vi "Vista superior.vi"() -> ()   [LabVIEW 2024]
uses:
  Lamborghini.v2.ctl
  Tsuru.ctl
  Enum. Estarcionar.ctl
  <vilib>/Utility/miscctls.llb/LVPositionTypeDef.ctl
panel:
  out "Retroceder 2":bool
  out "Estacionarse 2":bool
  out "Estacionarse":bool
  out "Retroceder":bool
  in  "Aparecer carro":bool
  in  "Carro":i32
  in  "F1 Auto":T1
  out "Pluma 3":u8(slide)
  out "Led 2":bool
  in  "Stop Button 3":bool
  in  "Tsuru":T2
  out "Pluma 2":u8(slide)
  out "Led 0":bool
  in  "Stop Button 2":bool
  in  "Lamborghini":T3
  out "Led 1":bool
  in  "Stop Button":bool
  out "Pluma":u8(slide)
  # "En el punto de la pluma se debe ver la\nanimación de la pluma levantándose."
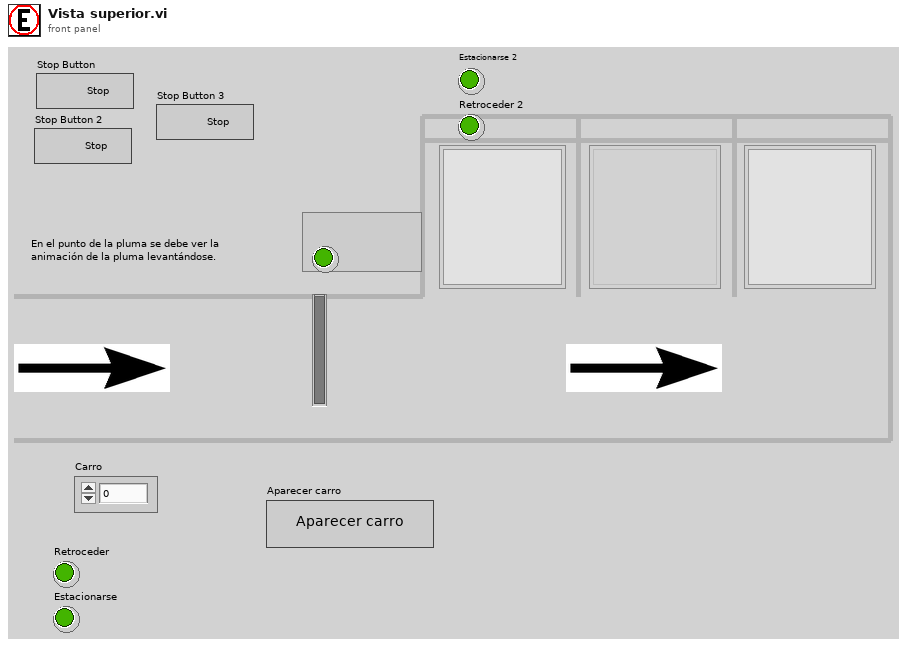
[diagram p1: front panel]
types:
  T1 = typedef "Fórmula 1.ctl" = u16
  T2 = typedef "Tsuru.ctl" = u16
  T3 = typedef "Lamborghini.v2.ctl" = u16
  T4 = typedef "Enum. Estarcionar.ctl" = enum16{"Llegar", "Acceso", "Retroceder", "Animación", "Pluma", "Avanzar", "Girar", "Estacionar", "No hacer nada"}
  T5 = typedef "LVPositionTypeDef.ctl" = cluster{"Left":i32, "Top":i32}
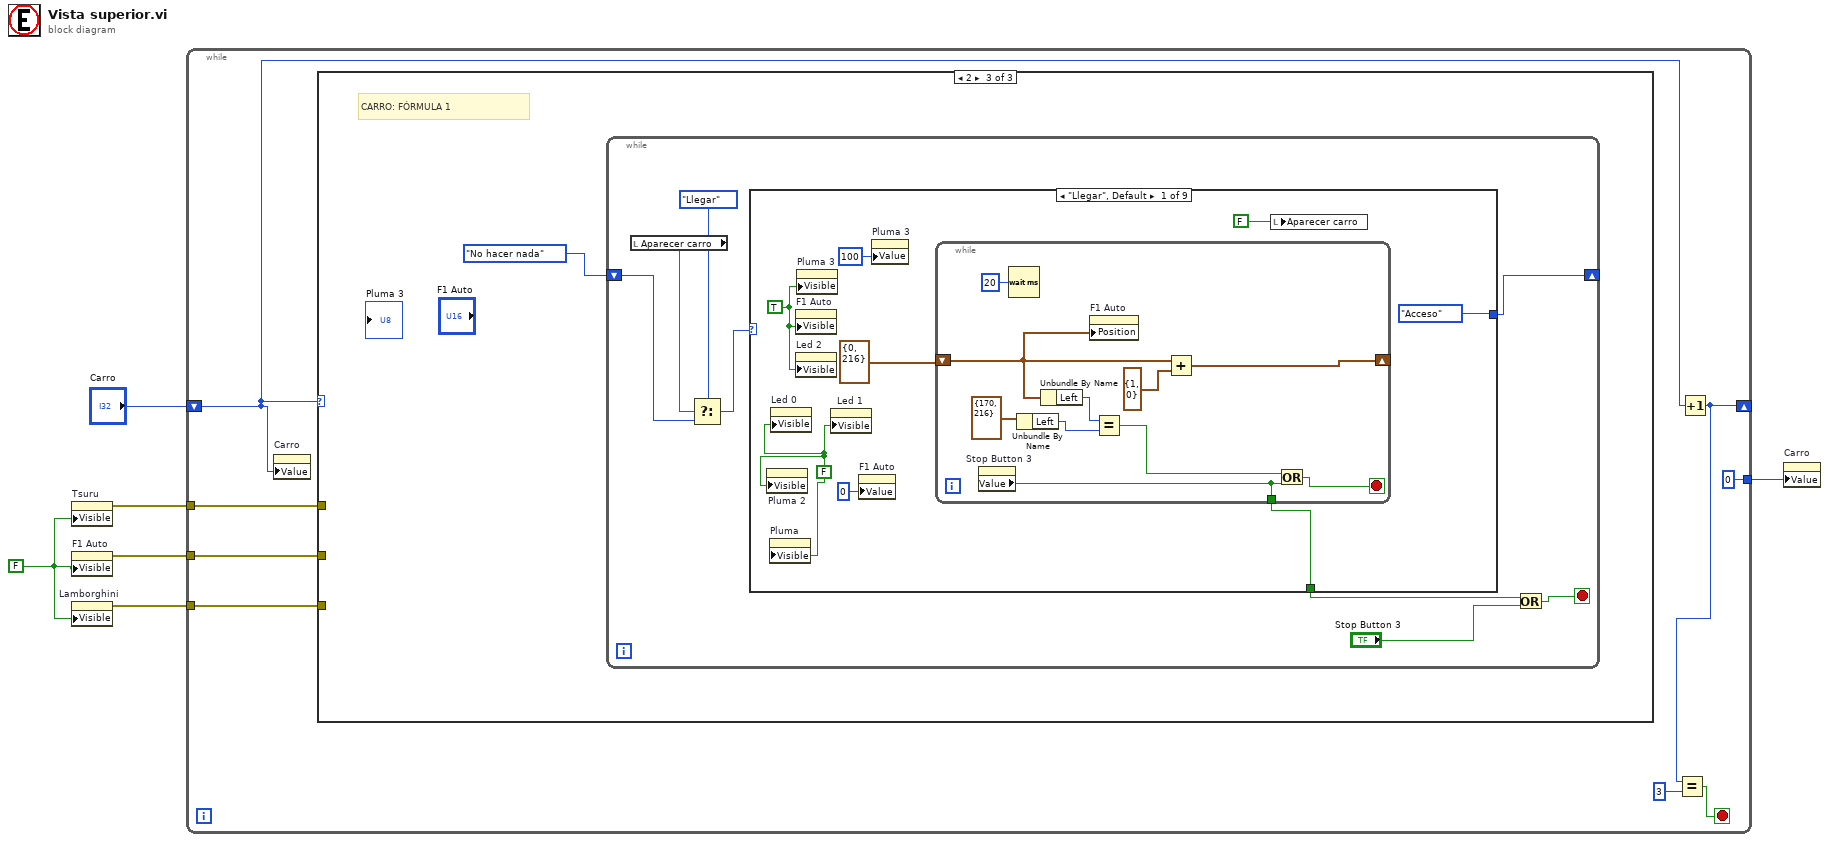
[diagram p0: block diagram]
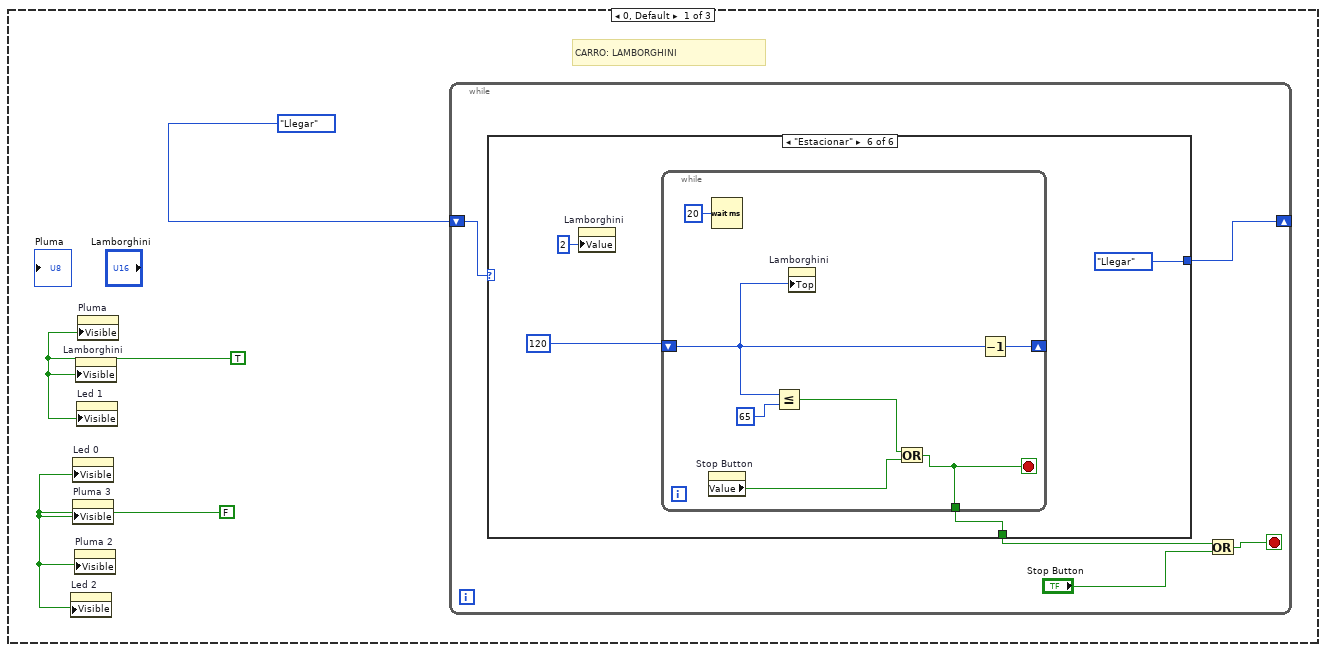
[diagram p2: hidden frame]
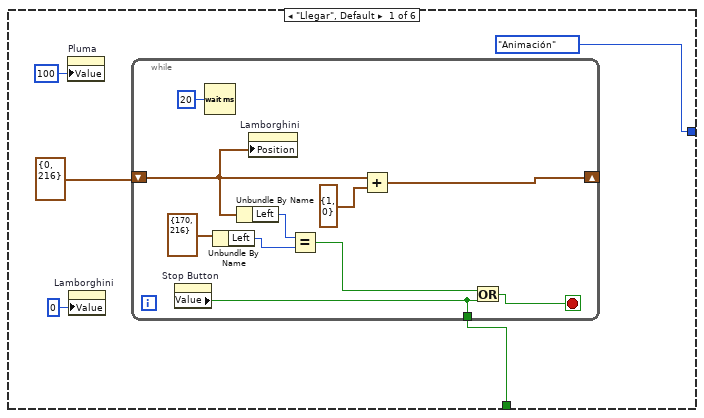
[diagram p3: hidden frame]
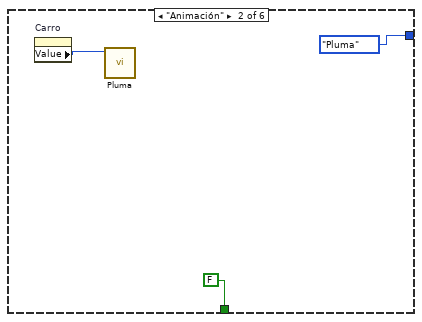
[diagram p4: hidden frame]
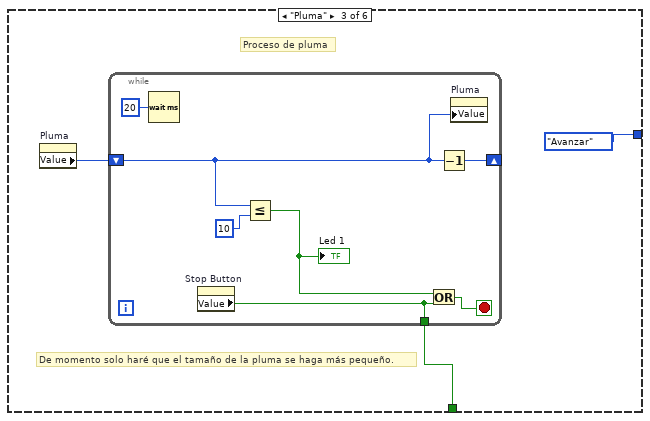
[diagram p5: hidden frame]
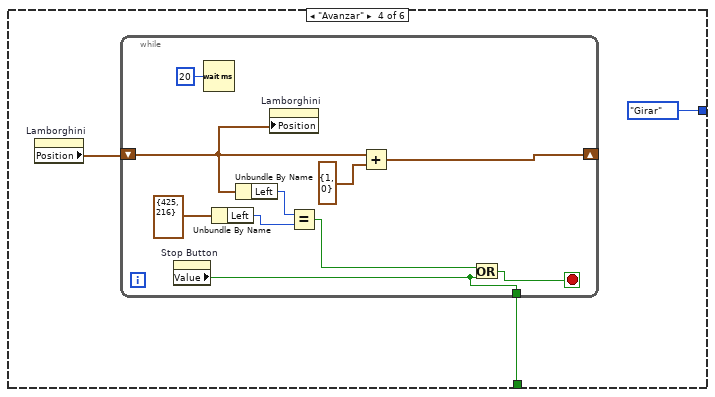
[diagram p6: hidden frame]
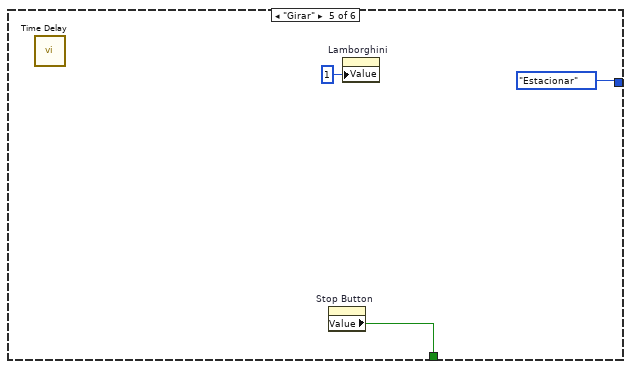
[diagram p7: hidden frame]
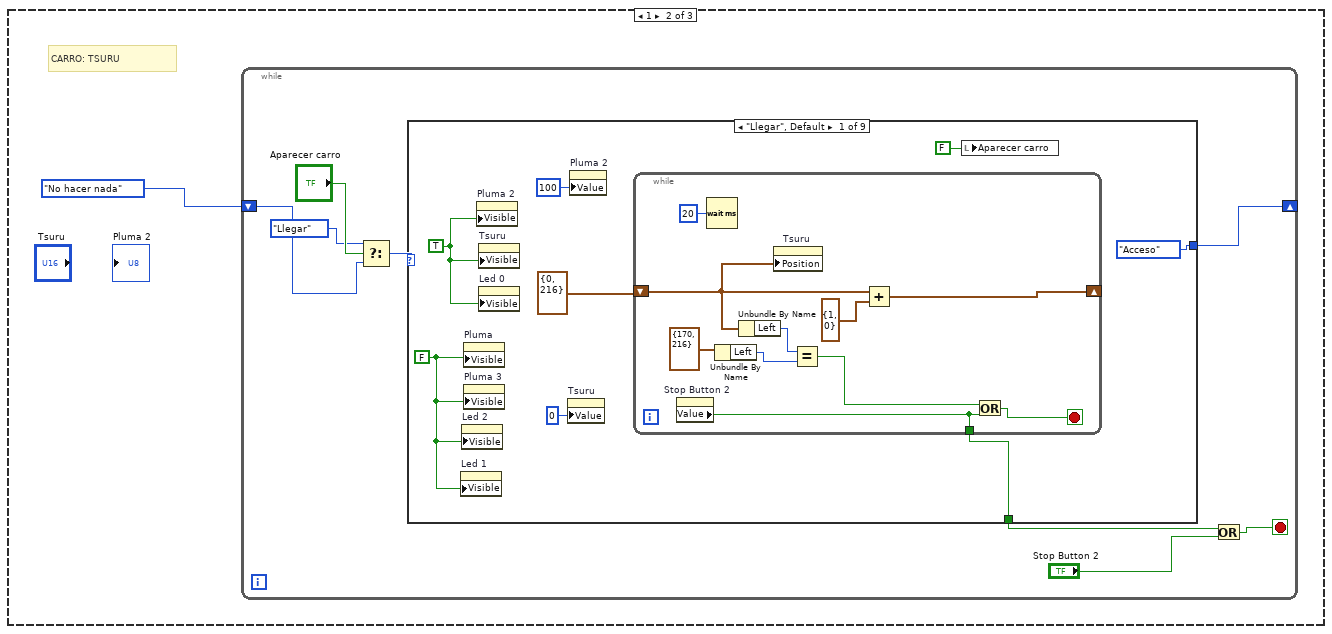
[diagram p8: hidden frame]
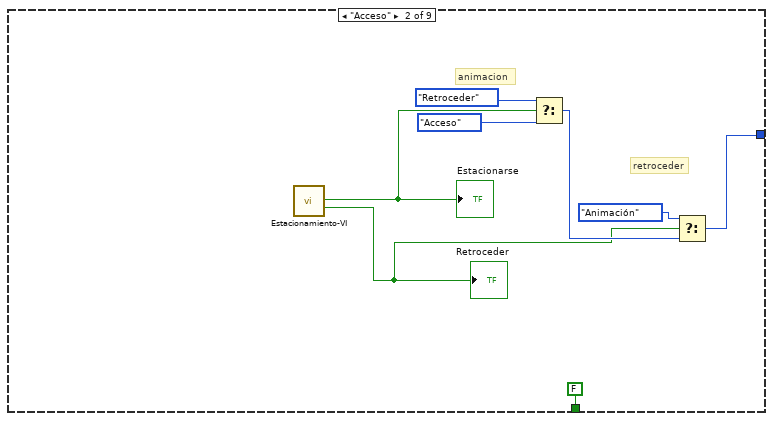
[diagram p9: hidden frame]
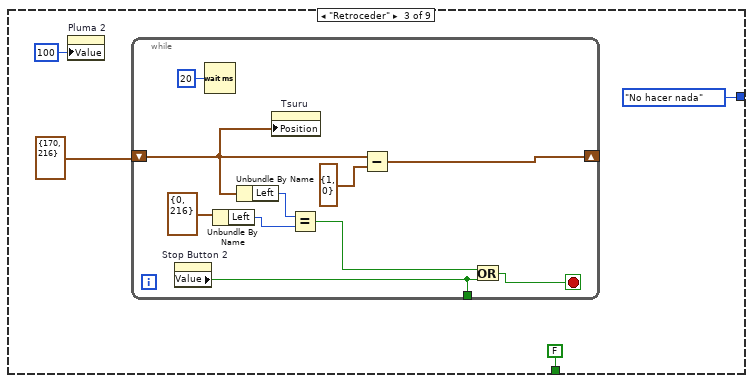
[diagram p10: hidden frame]
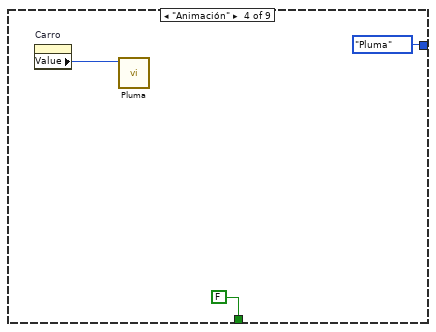
[diagram p11: hidden frame]
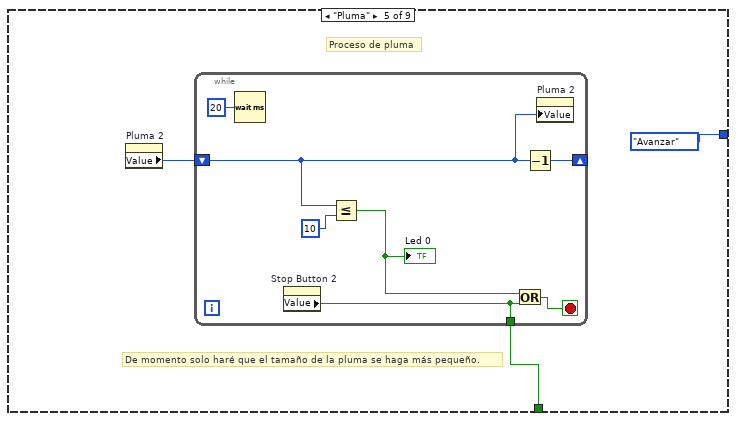
[diagram p12: hidden frame]
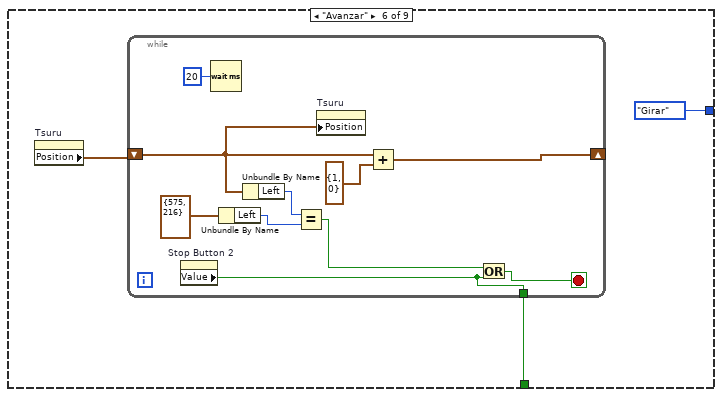
[diagram p13: hidden frame]
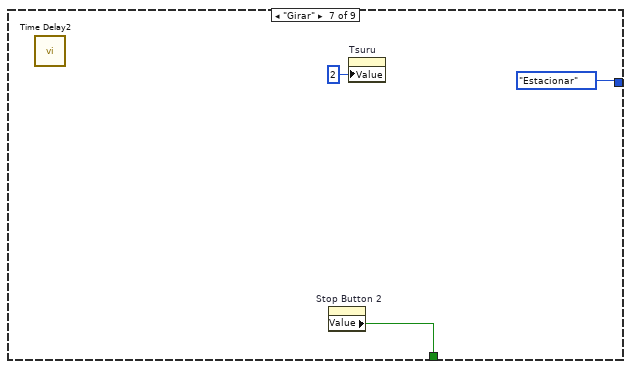
[diagram p14: hidden frame]
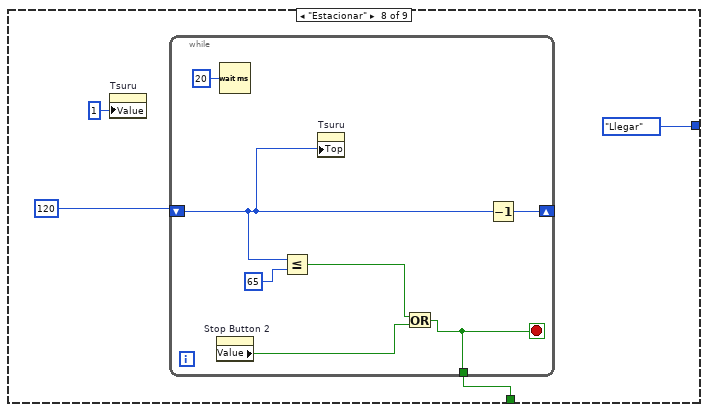
[diagram p15: hidden frame]
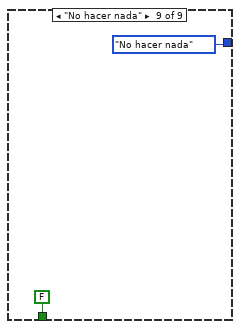
[diagram p16: hidden frame]
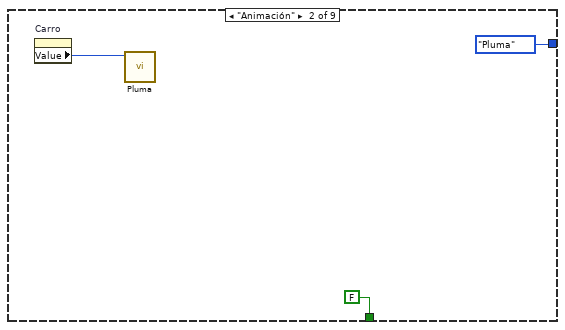
[diagram p17: hidden frame]
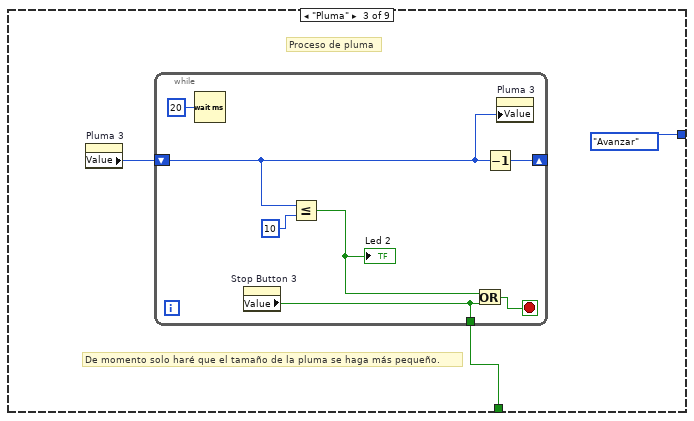
[diagram p18: hidden frame]
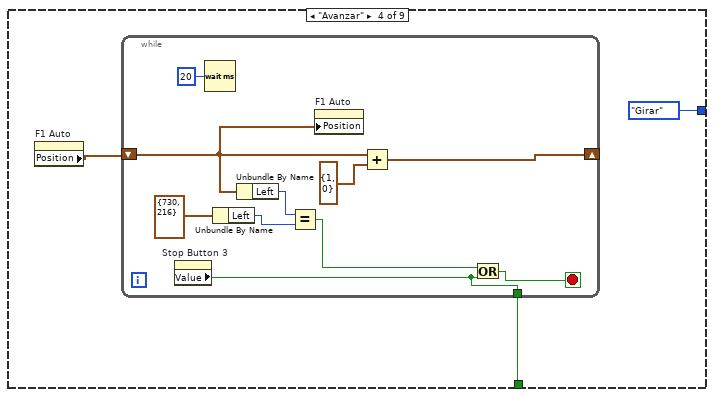
[diagram p19: hidden frame]
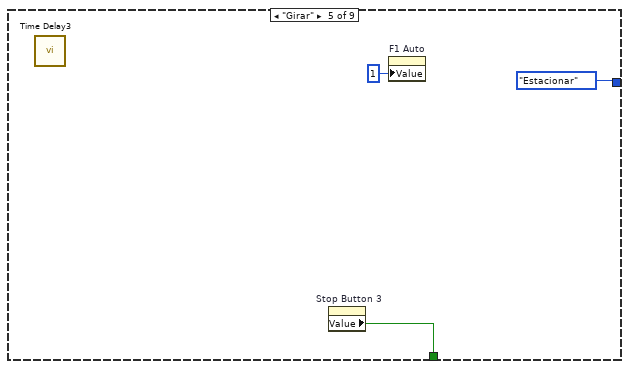
[diagram p20: hidden frame]
diagram:
  w3 = FALSE ("Visible")
  n1 = property on="Tsuru" class="Ring (strict)"("Visible"=w3) -> (error out=w6:errorcluster)  [unwired: 2 in, 1 out]
  n2 = property on="F1 Auto" class="Ring (strict)"("Visible"=w3) -> (error out=w5:errorcluster)  [unwired: 2 in, 1 out]
  n3 = property on="Lamborghini" class="Ring (strict)"("Visible"=w3) -> (error out=w4:errorcluster)  [unwired: 2 in, 1 out]
  n4 = while {
    tunnel: w6 -> [w14]
    tunnel: w5 -> [w13]
    tunnel: w4 -> [w12]
    shift-right: [w8] -> _
    shift-left: "Carro" -> [w7]
    tunnel: [0 ("Carro")] -> w1
    stop <- w11 stop-if-true
    n5 = property on="Carro" class="DigNum (strict)"("Value"=w7) -> ()  [unwired: 2 in, 2 out]
    n6 = case shown="2" w7 {
      tunnel: w14 -> [_ _ _]
      tunnel: w13 -> [_ _ _]
      tunnel: w12 -> [_ _ _]
      frame 0, Default {
        w16 = TRUE
        w15 = FALSE
        # "CARRO: LAMBORGHINI"
        n7 = property on="Led 2" class="Bool (strict)"("Visible"=w15) -> ()  [unwired: 2 in, 2 out]
        n8 = property on="Led 0" class="Bool (strict)"("Visible"=w15) -> ()  [unwired: 2 in, 2 out]
        n9 = property on="Pluma 3" class="Slide (strict)"("Visible"=w15) -> ()  [unwired: 2 in, 2 out]
        n10 = property on="Pluma 2" class="Slide (strict)"("Visible"=w15) -> ()  [unwired: 2 in, 2 out]
        n11 = property on="Lamborghini" class="Ring (strict)"("Visible"=w16) -> ()  [unwired: 2 in, 2 out]
        n12 = property on="Led 1" class="Bool (strict)"("Visible"=w16) -> ()  [unwired: 2 in, 2 out]
        n13 = property on="Pluma" class="Slide (strict)"("Visible"=w16) -> ()  [unwired: 2 in, 2 out]
        n14 = while {
          shift-right: [w21] -> _
          shift-left: Enum._Estarcionar."Llegar" -> [w22]
          stop <- w18 stop-if-true
          n15 = case shown="\"Estacionar\"" w22 {
            tunnel: [Enum._Estarcionar."Animación" Enum._Estarcionar."Pluma" Enum._Estarcionar."Avanzar" Enum._Estarcionar."Girar" Enum._Estarcionar."Estacionar" Enum._Estarcionar."Llegar"] -> w21
            tunnel: [w26 FALSE w42 w52 w65 w68] -> w19
            frame "Llegar", Default {
              n16 = property on="Pluma" class="Slide (strict)"("Value"=u8 100 ("Pluma")) -> ()  [unwired: 2 in, 2 out]
              n17 = property on="Lamborghini" class="Ring (strict)"("Value"=T3 0 ("Ring")) -> ()  [unwired: 2 in, 2 out]
              n18 = while {
                shift-right: [w31] -> _
                shift-left: T5 {"Left"=0, "Top"=216} ("y") -> [w28]
                tunnel: [w29] -> w26
                stop <- w30 stop-if-true
                n19 = property on="Stop Button" class="Bool (strict)"() -> ("Value"=w29:bool)  [unwired: 2 in, 2 out]
                n20 = Wait (ms)(milliseconds to wait=u32 20) -> ()  [unwired: 1 out]
                n21 = Unbundle By Name(T5 {"Left"=170, "Top"=216} ("y")) -> ("Left"=w33:i32)
                n22 = Unbundle By Name(w28) -> ("Left"=w32:i32)
                n23 = property on="Lamborghini" class="Ring (strict)"("Position"=w28) -> ()  [unwired: 2 in, 2 out]
                n24 = Equal?(x=w32, y=w33) -> (x = y?=w35:bool)
                n25 = Add(x=w28, y=T5 {"Left"=1, "Top"=0}) -> (x+y=w31:T5)
                n26 = Or(x=w35, y=w29) -> (x .or. y?=w30:bool)
              }
            }
            frame "Animación" {
              n27 = property on="Carro" class="DigNum (strict)"() -> ("Value"=w38:i32)  [unwired: 2 in, 2 out]
              n28 = call "Pluma.vi"("Numeric"=w38) -> ()  [unwired: 11 in]
            }
            frame "Pluma" {
              # "De momento solo haré que el tamaño de la pluma se haga más pequeño."
              # "Proceso de pluma"
              n29 = property on="Pluma" class="Slide (strict)"() -> ("Value"=w43:u8)  [unwired: 2 in, 2 out]
              n30 = while {
                shift-right: [w50] -> _
                shift-left: w43 -> [w48]
                tunnel: [w44] -> w42
                stop <- w45 stop-if-true
                n31 = Wait (ms)(milliseconds to wait=u32 20) -> ()  [unwired: 1 out]
                n32 = property on="Stop Button" class="Bool (strict)"() -> ("Value"=w44:bool)  [unwired: 2 in, 2 out]
                n33 = Less Or Equal?(x=w48, y=u8 10) -> (x <= y?=w46:bool)
                "Led 1" <- w46
                n34 = Or(x=w46, y=w44) -> (x .or. y?=w45:bool)
                n35 = Decrement(x=w48) -> (x-1=w50:u8)
                n36 = property on="Pluma" class="Slide (strict)"("Value"=w48) -> ()  [unwired: 2 in, 2 out]
              }
            }
            frame "Avanzar" {
              n37 = property on="Lamborghini" class="Ring (strict)"() -> ("Position"=w51:T5)  [unwired: 2 in, 2 out]
              n38 = while {
                shift-right: [w59] -> _
                shift-left: w51 -> [w55]
                tunnel: [w56] -> w52
                stop <- w58 stop-if-true
                n39 = property on="Stop Button" class="Bool (strict)"() -> ("Value"=w56:bool)  [unwired: 2 in, 2 out]
                n40 = Wait (ms)(milliseconds to wait=u32 20) -> ()  [unwired: 1 out]
                n41 = Unbundle By Name(T5 {"Left"=425, "Top"=216} ("input cluster")) -> ("Left"=w61:i32)
                n42 = Unbundle By Name(w55) -> ("Left"=w60:i32)
                n43 = property on="Lamborghini" class="Ring (strict)"("Position"=w55) -> ()  [unwired: 2 in, 2 out]
                n44 = Equal?(x=w60, y=w61) -> (x = y?=w57:bool)
                n45 = Add(x=w55, y=T5 {"Left"=1, "Top"=0}) -> (x+y=w59:T5)
                n46 = Or(x=w57, y=w56) -> (x .or. y?=w58:bool)
              }
            }
            frame "Girar" {
              n47 = call "Time Delay"() -> ()  [unwired: 11 in, 1 out]
              n48 = property on="Stop Button" class="Bool (strict)"() -> ("Value"=w65:bool)  [unwired: 2 in, 2 out]
              n49 = property on="Lamborghini" class="Ring (strict)"("Value"=T3 1 ("Ring")) -> ()  [unwired: 2 in, 2 out]
            }
            frame "Estacionar" {
              n50 = property on="Lamborghini" class="Ring (strict)"("Value"=T3 2 ("Ring")) -> ()  [unwired: 2 in, 2 out]
              n51 = while {
                shift-right: [w77] -> _
                shift-left: 120 ("Top") -> [w73]
                tunnel: [w71] -> w68
                stop <- w71 stop-if-true
                n52 = property on="Stop Button" class="Bool (strict)"() -> ("Value"=w72:bool)  [unwired: 2 in, 2 out]
                n53 = Wait (ms)(milliseconds to wait=u32 20) -> ()  [unwired: 1 out]
                n54 = Less Or Equal?(x=w73, y=65) -> (x <= y?=w74:bool)
                n55 = property on="Lamborghini" class="Ring (strict)"("Top"=w73) -> ()  [unwired: 2 in, 2 out]
                n56 = Or(x=w74, y=w72) -> (x .or. y?=w71:bool)
                n57 = Decrement(x=w73) -> (x-1=w77:i32)
              }
            }
          }
          n58 = Or(x=w19, y="Stop Button") -> (x .or. y?=w18:bool)
        }
      }
      frame 1 {
        # "CARRO: TSURU"
        n59 = while {
          shift-right: [w86] -> _
          shift-left: Enum._Estarcionar."No hacer nada" -> [w79]
          stop <- w83 stop-if-true
          n60 = Select(t=Enum._Estarcionar."Llegar", s="Aparecer carro", f=w79) -> (s? t:f=w80:T4)
          n61 = case shown="\"Llegar\", Default" w80 {
            tunnel: [Enum._Estarcionar."Acceso" w108 Enum._Estarcionar."No hacer nada" Enum._Estarcionar."Pluma" Enum._Estarcionar."Avanzar" Enum._Estarcionar."Girar" Enum._Estarcionar."Estacionar" Enum._Estarcionar."Llegar" Enum._Estarcionar."No hacer nada"] -> w86
            tunnel: [w93 FALSE ("Value") FALSE ("Value") FALSE w131 w141 w154 w157 FALSE ("Value")] -> w84
            frame "Llegar", Default {
              w88 = TRUE
              w89 = FALSE
              n62 = property on="Led 1" class="Bool (strict)"("Visible"=w89) -> ()  [unwired: 2 in, 2 out]
              n63 = property on="Led 2" class="Bool (strict)"("Visible"=w89) -> ()  [unwired: 2 in, 2 out]
              n64 = property on="Pluma" class="Slide (strict)"("Visible"=w89) -> ()  [unwired: 2 in, 2 out]
              n65 = property on="Pluma 3" class="Slide (strict)"("Visible"=w89) -> ()  [unwired: 2 in, 2 out]
              n66 = property on="Pluma 2" class="Slide (strict)"("Visible"=w88) -> ()  [unwired: 2 in, 2 out]
              n67 = property on="Tsuru" class="Ring (strict)"("Visible"=w88) -> ()  [unwired: 2 in, 2 out]
              n68 = property on="Led 0" class="Bool (strict)"("Visible"=w88) -> ()  [unwired: 2 in, 2 out]
              n69 = property on="Tsuru" class="Ring (strict)"("Value"=T2 0 ("Tsuru")) -> ()  [unwired: 2 in, 2 out]
              n70 = property on="Pluma 2" class="Slide (strict)"("Value"=u8 100 ("Pluma")) -> ()  [unwired: 2 in, 2 out]
              n71 = while {
                shift-right: [w98] -> _
                shift-left: T5 {"Left"=0, "Top"=216} ("y") -> [w95]
                tunnel: [w96] -> w93
                stop <- w97 stop-if-true
                n72 = property on="Stop Button 2" class="Bool (strict)"() -> ("Value"=w96:bool)  [unwired: 2 in, 2 out]
                n73 = Wait (ms)(milliseconds to wait=u32 20) -> ()  [unwired: 1 out]
                n74 = Unbundle By Name(T5 {"Left"=170, "Top"=216} ("y")) -> ("Left"=w100:i32)
                n75 = Unbundle By Name(w95) -> ("Left"=w99:i32)
                n76 = property on="Tsuru" class="Ring (strict)"("Position"=w95) -> ()  [unwired: 2 in, 2 out]
                n77 = Equal?(x=w99, y=w100) -> (x = y?=w102:bool)
                n78 = Add(x=w95, y=T5 {"Left"=1, "Top"=0}) -> (x+y=w98:T5)
                n79 = Or(x=w102, y=w96) -> (x .or. y?=w97:bool)
              }
              n80 = local write "Aparecer carro"(FALSE) -> ()
            }
            frame "Acceso" {
              # "retroceder"
              # "animacion"
              n81 = call "Estacionamiento-VI.vi"() -> ("Estacionarse"=w106:bool, "Retroceder"=w105:bool)  [unwired: 8 in]
              "Retroceder" <- w105
              "Estacionarse" <- w106
              n82 = Select(t=Enum._Estarcionar."Retroceder", s=w106, f=Enum._Estarcionar."Acceso") -> (s? t:f=w109:T4)
              n83 = Select(t=Enum._Estarcionar."Animación", s=w105, f=w109) -> (s? t:f=w108:T4)
            }
            frame "Retroceder" {
              n84 = property on="Pluma 2" class="Slide (strict)"("Value"=u8 100 ("Pluma")) -> ()  [unwired: 2 in, 2 out]
              n85 = while {
                shift-right: [w120] -> _
                shift-left: T5 {"Left"=170, "Top"=216} ("y") -> [w117]
                tunnel: [w118] -> _
                stop <- w119 stop-if-true
                n86 = property on="Stop Button 2" class="Bool (strict)"() -> ("Value"=w118:bool)  [unwired: 2 in, 2 out]
                n87 = Wait (ms)(milliseconds to wait=u32 20) -> ()  [unwired: 1 out]
                n88 = Unbundle By Name(T5 {"Left"=0, "Top"=216} ("y")) -> ("Left"=w122:i32)
                n89 = Unbundle By Name(w117) -> ("Left"=w121:i32)
                n90 = property on="Tsuru" class="Ring (strict)"("Position"=w117) -> ()  [unwired: 2 in, 2 out]
                n91 = Equal?(x=w121, y=w122) -> (x = y?=w124:bool)
                n92 = Subtract(x=w117, y=T5 {"Left"=1, "Top"=0}) -> (x-y=w120:T5)
                n93 = Or(x=w124, y=w118) -> (x .or. y?=w119:bool)
              }
            }
            frame "Animación" {
              n94 = property on="Carro" class="DigNum (strict)"() -> ("Value"=w127:i32)  [unwired: 2 in, 2 out]
              n95 = call "Pluma.vi"("Numeric"=w127) -> ()  [unwired: 11 in]
            }
            frame "Pluma" {
              # "De momento solo haré que el tamaño de la pluma se haga más pequeño."
              # "Proceso de pluma"
              n96 = property on="Pluma 2" class="Slide (strict)"() -> ("Value"=w132:u8)  [unwired: 2 in, 2 out]
              n97 = while {
                shift-right: [w139] -> _
                shift-left: w132 -> [w137]
                tunnel: [w133] -> w131
                stop <- w134 stop-if-true
                n98 = Wait (ms)(milliseconds to wait=u32 20) -> ()  [unwired: 1 out]
                n99 = property on="Stop Button 2" class="Bool (strict)"() -> ("Value"=w133:bool)  [unwired: 2 in, 2 out]
                n100 = Less Or Equal?(x=w137, y=u8 10) -> (x <= y?=w135:bool)
                "Led 0" <- w135
                n101 = Or(x=w135, y=w133) -> (x .or. y?=w134:bool)
                n102 = Decrement(x=w137) -> (x-1=w139:u8)
                n103 = property on="Pluma 2" class="Slide (strict)"("Value"=w137) -> ()  [unwired: 2 in, 2 out]
              }
            }
            frame "Avanzar" {
              n104 = property on="Tsuru" class="Ring (strict)"() -> ("Position"=w140:T5)  [unwired: 2 in, 2 out]
              n105 = while {
                shift-right: [w148] -> _
                shift-left: w140 -> [w143]
                tunnel: [w145] -> w141
                stop <- w147 stop-if-true
                n106 = property on="Stop Button 2" class="Bool (strict)"() -> ("Value"=w145:bool)  [unwired: 2 in, 2 out]
                n107 = Wait (ms)(milliseconds to wait=u32 20) -> ()  [unwired: 1 out]
                n108 = Unbundle By Name(T5 {"Left"=575, "Top"=216} ("input cluster")) -> ("Left"=w150:i32)
                n109 = Unbundle By Name(w143) -> ("Left"=w149:i32)
                n110 = Equal?(x=w149, y=w150) -> (x = y?=w146:bool)
                n111 = property on="Tsuru" class="Ring (strict)"("Position"=w143) -> ()  [unwired: 2 in, 2 out]
                n112 = Add(x=w143, y=T5 {"Left"=1, "Top"=0}) -> (x+y=w148:T5)
                n113 = Or(x=w146, y=w145) -> (x .or. y?=w147:bool)
              }
            }
            frame "Girar" {
              n114 = call "Time Delay2"() -> ()  [unwired: 11 in, 1 out]
              n115 = property on="Stop Button 2" class="Bool (strict)"() -> ("Value"=w154:bool)  [unwired: 2 in, 2 out]
              n116 = property on="Tsuru" class="Ring (strict)"("Value"=T2 2 ("Tsuru")) -> ()  [unwired: 2 in, 2 out]
            }
            frame "Estacionar" {
              n117 = property on="Tsuru" class="Ring (strict)"("Value"=T2 1 ("Tsuru")) -> ()  [unwired: 2 in, 2 out]
              n118 = while {
                shift-right: [w166] -> _
                shift-left: 120 ("Top") -> [w162]
                tunnel: [w160] -> w157
                stop <- w160 stop-if-true
                n119 = property on="Stop Button 2" class="Bool (strict)"() -> ("Value"=w161:bool)  [unwired: 2 in, 2 out]
                n120 = Wait (ms)(milliseconds to wait=u32 20) -> ()  [unwired: 1 out]
                n121 = Less Or Equal?(x=w162, y=65) -> (x <= y?=w163:bool)
                n122 = property on="Tsuru" class="Ring (strict)"("Top"=w162) -> ()  [unwired: 2 in, 2 out]
                n123 = Or(x=w163, y=w161) -> (x .or. y?=w160:bool)
                n124 = Decrement(x=w162) -> (x-1=w166:i32)
              }
            }
            frame "No hacer nada" {
            }
          }
          n125 = Or(x=w84, y="Stop Button 2") -> (x .or. y?=w83:bool)
        }
      }
      frame 2 {
        # "CARRO: FÓRMULA 1"
        n126 = while {
          shift-right: [w177] -> _
          shift-left: Enum._Estarcionar."No hacer nada" -> [w170]
          stop <- w174 stop-if-true
          n127 = local read "Aparecer carro"() -> (w171:bool)
          n128 = Select(t=Enum._Estarcionar."Llegar", s=w171, f=w170) -> (s? t:f=w172:T4)
          n129 = case shown="\"Llegar\", Default" w172 {
            tunnel: [Enum._Estarcionar."Acceso" Enum._Estarcionar."Pluma" Enum._Estarcionar."Avanzar" Enum._Estarcionar."Girar" Enum._Estarcionar."Estacionar" Enum._Estarcionar."Llegar" Enum._Estarcionar."No hacer nada" w238 Enum._Estarcionar."No hacer nada"] -> w177
            tunnel: [w183 FALSE w200 w210 w223 w226 FALSE FALSE FALSE] -> w175
            frame "Llegar", Default {
              w179 = TRUE
              w180 = FALSE
              n130 = property on="Pluma 2" class="Slide (strict)"("Visible"=w180) -> ()  [unwired: 2 in, 2 out]
              n131 = property on="Pluma" class="Slide (strict)"("Visible"=w180) -> ()  [unwired: 2 in, 2 out]
              n132 = property on="Led 0" class="Bool (strict)"("Visible"=w180) -> ()  [unwired: 2 in, 2 out]
              n133 = property on="F1 Auto" class="Ring (strict)"("Visible"=w179) -> ()  [unwired: 2 in, 2 out]
              n134 = property on="Led 2" class="Bool (strict)"("Visible"=w179) -> ()  [unwired: 2 in, 2 out]
              n135 = property on="Pluma 3" class="Slide (strict)"("Visible"=w179) -> ()  [unwired: 2 in, 2 out]
              n136 = property on="Led 1" class="Bool (strict)"("Visible"=w180) -> ()  [unwired: 2 in, 2 out]
              n137 = property on="F1 Auto" class="Ring (strict)"("Value"=T1 0 ("F1 Auto")) -> ()  [unwired: 2 in, 2 out]
              n138 = property on="Pluma 3" class="Slide (strict)"("Value"=u8 100 ("Pluma")) -> ()  [unwired: 2 in, 2 out]
              n139 = while {
                shift-right: [w189] -> _
                shift-left: T5 {"Left"=0, "Top"=216} ("y") -> [w186]
                tunnel: [w187] -> w183
                stop <- w188 stop-if-true
                n140 = property on="Stop Button 3" class="Bool (strict)"() -> ("Value"=w187:bool)  [unwired: 2 in, 2 out]
                n141 = Wait (ms)(milliseconds to wait=u32 20) -> ()  [unwired: 1 out]
                n142 = Unbundle By Name(T5 {"Left"=170, "Top"=216} ("y")) -> ("Left"=w191:i32)
                n143 = Unbundle By Name(w186) -> ("Left"=w190:i32)
                n144 = property on="F1 Auto" class="Ring (strict)"("Position"=w186) -> ()  [unwired: 2 in, 2 out]
                n145 = Equal?(x=w190, y=w191) -> (x = y?=w193:bool)
                n146 = Add(x=w186, y=T5 {"Left"=1, "Top"=0}) -> (x+y=w189:T5)
                n147 = Or(x=w193, y=w187) -> (x .or. y?=w188:bool)
              }
              n148 = local write "Aparecer carro"(FALSE) -> ()
            }
            frame "Animación" {
              n149 = property on="Carro" class="DigNum (strict)"() -> ("Value"=w196:i32)  [unwired: 2 in, 2 out]
              n150 = call "Pluma.vi"("Numeric"=w196) -> ()  [unwired: 11 in]
            }
            frame "Pluma" {
              # "De momento solo haré que el tamaño de la pluma se haga más pequeño."
              # "Proceso de pluma"
              n151 = property on="Pluma 3" class="Slide (strict)"() -> ("Value"=w201:u8)  [unwired: 2 in, 2 out]
              n152 = while {
                shift-right: [w208] -> _
                shift-left: w201 -> [w206]
                tunnel: [w202] -> w200
                stop <- w203 stop-if-true
                n153 = Wait (ms)(milliseconds to wait=u32 20) -> ()  [unwired: 1 out]
                n154 = property on="Stop Button 3" class="Bool (strict)"() -> ("Value"=w202:bool)  [unwired: 2 in, 2 out]
                n155 = Less Or Equal?(x=w206, y=u8 10) -> (x <= y?=w204:bool)
                "Led 2" <- w204
                n156 = Or(x=w204, y=w202) -> (x .or. y?=w203:bool)
                n157 = Decrement(x=w206) -> (x-1=w208:u8)
                n158 = property on="Pluma 3" class="Slide (strict)"("Value"=w206) -> ()  [unwired: 2 in, 2 out]
              }
            }
            frame "Avanzar" {
              n159 = property on="F1 Auto" class="Ring (strict)"() -> ("Position"=w209:T5)  [unwired: 2 in, 2 out]
              n160 = while {
                shift-right: [w217] -> _
                shift-left: w209 -> [w212]
                tunnel: [w214] -> w210
                stop <- w216 stop-if-true
                n161 = property on="Stop Button 3" class="Bool (strict)"() -> ("Value"=w214:bool)  [unwired: 2 in, 2 out]
                n162 = Wait (ms)(milliseconds to wait=u32 20) -> ()  [unwired: 1 out]
                n163 = Unbundle By Name(T5 {"Left"=730, "Top"=216} ("input cluster")) -> ("Left"=w219:i32)
                n164 = Unbundle By Name(w212) -> ("Left"=w218:i32)
                n165 = Equal?(x=w218, y=w219) -> (x = y?=w215:bool)
                n166 = property on="F1 Auto" class="Ring (strict)"("Position"=w212) -> ()  [unwired: 2 in, 2 out]
                n167 = Add(x=w212, y=T5 {"Left"=1, "Top"=0}) -> (x+y=w217:T5)
                n168 = Or(x=w215, y=w214) -> (x .or. y?=w216:bool)
              }
            }
            frame "Girar" {
              n169 = call "Time Delay3"() -> ()  [unwired: 11 in, 1 out]
              n170 = property on="Stop Button 3" class="Bool (strict)"() -> ("Value"=w223:bool)  [unwired: 2 in, 2 out]
              n171 = property on="F1 Auto" class="Ring (strict)"("Value"=T1 1 ("F1 Auto")) -> ()  [unwired: 2 in, 2 out]
            }
            frame "Estacionar" {
              n172 = property on="F1 Auto" class="Ring (strict)"("Value"=T1 2 ("F1 Auto")) -> ()  [unwired: 2 in, 2 out]
              n173 = while {
                shift-right: [w235] -> _
                shift-left: 120 ("Top") -> [w231]
                tunnel: [w229] -> w226
                stop <- w229 stop-if-true
                n174 = property on="Stop Button 3" class="Bool (strict)"() -> ("Value"=w230:bool)  [unwired: 2 in, 2 out]
                n175 = Wait (ms)(milliseconds to wait=u32 20) -> ()  [unwired: 1 out]
                n176 = property on="F1 Auto" class="Ring (strict)"("Top"=w231) -> ()  [unwired: 2 in, 2 out]
                n177 = Less Or Equal?(x=w231, y=65) -> (x <= y?=w232:bool)
                n178 = Or(x=w232, y=w230) -> (x .or. y?=w229:bool)
                n179 = Decrement(x=w231) -> (x-1=w235:i32)
              }
            }
            frame "No hacer nada" {
            }
            frame "Acceso" {
              # "retroceder"
              # "animacion"
              n180 = call "Estacionamiento-VI.vi"() -> ("Estacionarse"=w243:bool, "Retroceder"=w242:bool)  [unwired: 8 in]
              "Retroceder 2" <- w242
              "Estacionarse 2" <- w243
              n181 = Select(t=Enum._Estarcionar."Retroceder", s=w243, f=Enum._Estarcionar."Acceso") -> (s? t:f=w244:T4)
              n182 = Select(t=Enum._Estarcionar."Animación", s=w242, f=w244) -> (s? t:f=w238:T4)
            }
            frame "Retroceder" {
            }
          }
          n183 = Or(x=w175, y="Stop Button 3") -> (x .or. y?=w174:bool)
        }
      }
    }
    n184 = Increment(x=w7) -> (x+1=w8:i32)
    n185 = Equal?(x=w8, y=3) -> (x = y?=w11:bool)
  }
  n186 = property on="Carro" class="DigNum (strict)"("Value"=w1) -> ()  [unwired: 2 in, 2 out]
